vi "IPI_InitialCCD.vi"(8 "error in":errorcluster) -> (0 "error out":errorcluster, 3 "Session Out":T1)   [LabVIEW 2015]
uses:
  <vilib>/userdefined/High Color/IMAQdx.ctl
  <vilib>/vision/driver/NI_Vision_Acquisition_Software.lvlib
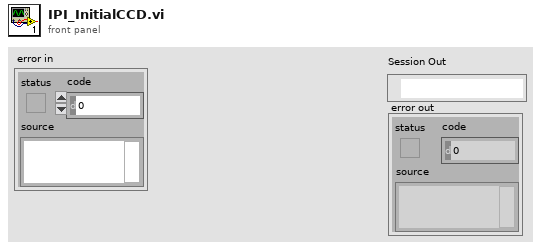
[diagram p1: front panel]
types:
  T1 = typedef "IMAQdx.ctl" = refnum<k21>
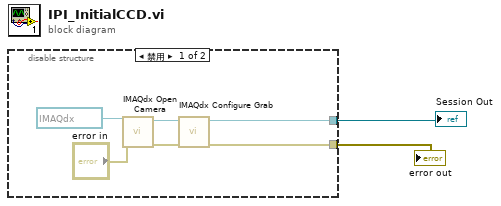
[diagram p0: block diagram]
diagram:
  n1 = disable-structure shown="禁用" {
    disable-tunnel: [w6 _] -> w2
    disable-tunnel: [w5 _] -> w1
    frame Disabled {
      n2 = call <vilib>:"IMAQdx Open Camera.vi"("error in"="error in", "Session In"=T1 "EXG50") -> ("error out"=w8:errorcluster, "Session Out"=w7:T1)  [unwired: 1 in, 7 out]
      n3 = call <vilib>:"IMAQdx Configure Grab.vi"("error in"=w8, "Session In"=w7) -> ("error out"=w5:errorcluster, "Session Out"=w6:T1)  [unwired: 8 out]
    }
    frame Enabled {
    }
  }
  "Session Out" <- w2
  "error out" <- w1
